vi "Set new direction.vi"(7 "Direction map":T2, 11 "Direction":T4) -> (3 "Direction Out":T4, 5 "Split Direction":T4)   [LabVIEW 2023]
uses:
  ENUM_Direction.ctl
  ENUM_Direction_a2.ctl
  Cluster_Point.ctl
  Map_Direction Next.ctl
panel:
  in  "Range":T1
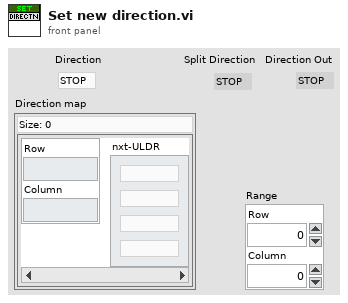
[diagram p1: front panel]
types:
  T1 = typedef "Cluster_Point.ctl" = cluster{"Row":i32, "Column":i32}
  T2 = typedef "Map_Direction Next.ctl" = map{T1, T3[]}
  T3 = typedef "ENUM_Direction_a2.ctl" = enum16{"Up", "Left", "Down", "Right", "Up-Down", "Left-Right"}
  T4 = typedef "ENUM_Direction.ctl" = enum16{"STOP", "Up", "Left", "Down", "Right"}
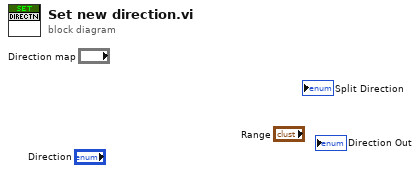
[diagram p0: block diagram]
diagram:
